vi "PowerControl.vi"(6 "Combo Box":string(combo), 9 "Voltage":string="1", 10 "Channel":string="1", 11 "address":string) -> (0 "error out":errorcluster)   [LabVIEW 2024]
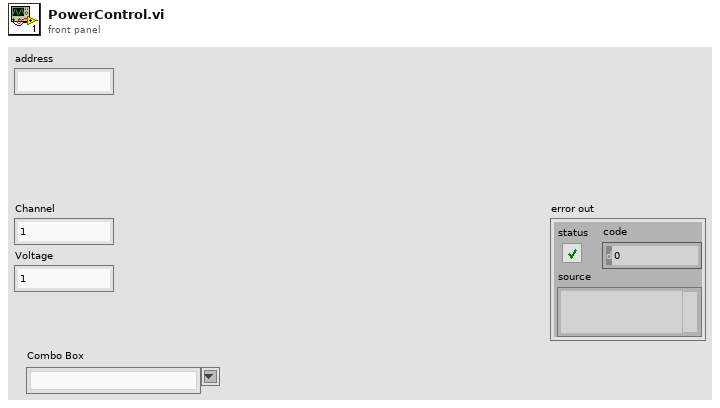
[diagram p1: front panel]
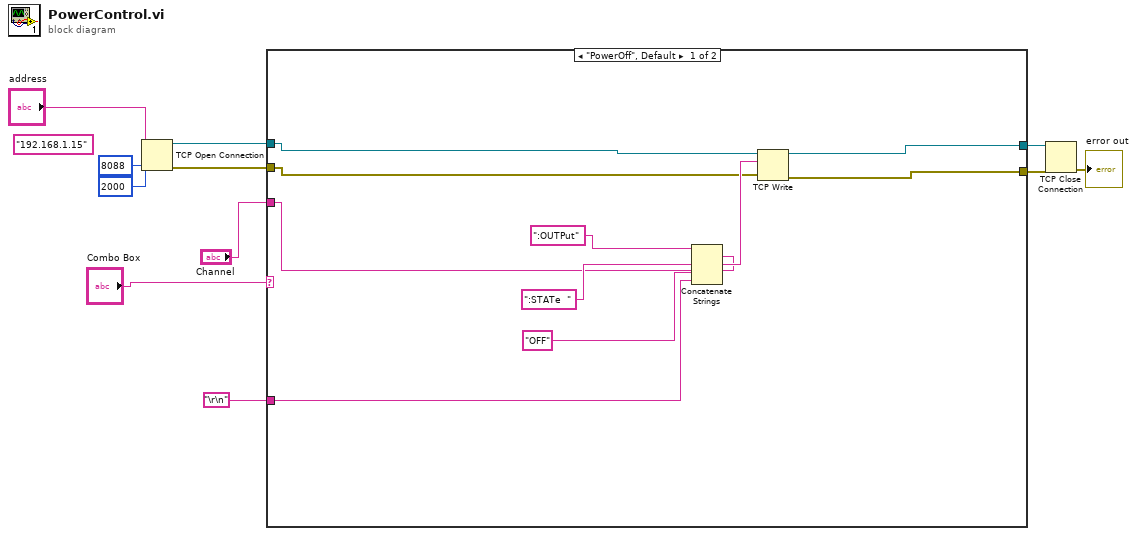
[diagram p0: block diagram]
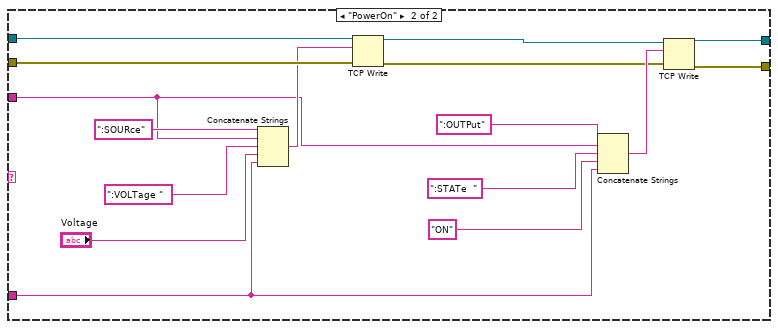
[diagram p2: hidden frame]
diagram:
  (unwired) "192.168.1.15" ("address")
  n1 = TCP Open Connection(address="address", remote port or service name=u16 8088, timeout ms (60000)=2000) -> (connection ID=w11:refnum<k5>, error out=w10:errorcluster)  [unwired: 2 in]
  n2 = case shown="\"PowerOff\", Default" "Combo Box" {
    tunnel: w11 -> [w17 w37]
    tunnel: w10 -> [w15 w36]
    tunnel: [w16 w25] -> w8
    tunnel: [w14 w24] -> w7
    tunnel: "Channel" -> [w13 w23]
    tunnel: "\r\n" -> [w12 w22]
    frame "PowerOff", Default {
      n3 = Concatenate Strings(":OUTPut", w13, ":STATe  ", "OFF", w12) -> (w21:string)
      n4 = TCP Write(connection ID=w17, data in=w21, error in (no error)=w15) -> (connection ID out=w16:refnum<k5>, error out=w14:errorcluster)  [unwired: 1 in, 1 out]
    }
    frame "PowerOn" {
      n5 = Concatenate Strings(":SOURce", w23, ":VOLTage ", "Voltage", w22) -> (w32:string)
      n6 = TCP Write(connection ID=w37, data in=w32, error in (no error)=w36) -> (connection ID out=w27:refnum<k5>, error out=w26:errorcluster)  [unwired: 1 in, 1 out]
      n7 = Concatenate Strings(":OUTPut", w23, ":STATe  ", "ON", w22) -> (w28:string)
      n8 = TCP Write(connection ID=w27, data in=w28, error in (no error)=w26) -> (connection ID out=w25:refnum<k5>, error out=w24:errorcluster)  [unwired: 1 in, 1 out]
    }
  }
  n9 = TCP Close Connection(connection ID=w8, error in (no error)=w7) -> (error out=→"error out":errorcluster)  [unwired: 1 in, 1 out]
